vi "Get File Length.vi"(0 "Filename":path) -> (4 "total number of samples/ch":u32, 15 "error out":errorcluster)   [LabVIEW 2020, in "File.lvclass"]
uses:
  File.lvclass
  <vilib>/sound2/lvsound2.llb/Sound File Info (path).vi
panel:
  in  "error in (no error)":errorcluster
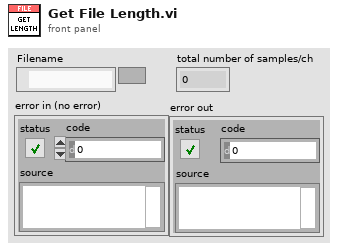
[diagram p1: front panel]
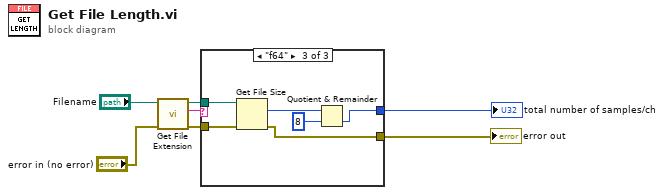
[diagram p0: block diagram]
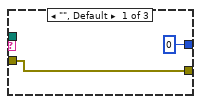
[diagram p2: hidden frame]
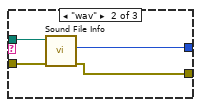
[diagram p3: hidden frame]
diagram:
  n1 = call <vilib>:"Get File Extension.vi"("error in (no error)"="error in (no error)", "file"="Filename") -> ("error out"=w2:errorcluster, "lowercase file extension"=w1:string, "dup file"=w4:path)  [unwired: 5 in, 2 out]
  n2 = case shown="\"f64\"" w1 {
    tunnel: [w8 w13 w14] -> w7
    tunnel: [u32 0 ("total number of samples/ch") w12 w16] -> w6
    tunnel: w4 -> [_ w11 w19]
    tunnel: w2 -> [w8 w10 w18]
    frame "", Default {
    }
    frame "wav" {
      n3 = call-poly <vilib>:"Sound File Info.vi"("error in (no error)"=w10, "path"=w11) -> ("error out"=w13:errorcluster, "total number of samples/ch"=w12:u32)  [unwired: 6 in, 2 out]
    }
    frame "f64" {
      n4 = Get File Size(file=w19, error in=w18) -> (size (in bytes)=w17:i64, 0:w14:errorcluster)  [unwired: 1 out]
      n5 = Quotient & Remainder(x=w17, y=i64 8) -> (floor(x/y)=w16:i64)  [unwired: 1 out]
    }
  }
  "error out" <- w7
  "total number of samples/ch" <- w6
